vi "PTC-Restore Defaults.vi"(11 "error in (no error)":errorcluster) -> (8 "Params":T1={"Ear"=enum."Right", "Stimulus"={"Type"="", "Freq step (Hz)"=50.0, "Sampling rate (Hz)"=50000.0, "Attenuation (dB)"=20.0}, "Averages"=0, "Cal Mic Gain"=0.0, "Probe Mic Gain"=0.0, "Cal Mic Sens"=0.0, "Correction"=path ""}, 15 "error out":errorcluster)   [LabVIEW 2020]
uses:
  Typedefs/PTC-Parameters.ctl
  Common VIs/Typedefs/CAL-Stimulus.ctl
  fdd48b6a-4494-43b2-9d05-00e0dea0306e.vi
  epl-vi-lib/Utility VIs/File IO VIs/Read Write Anything/Read Anything.vi
panel:
  in  "Defaults":T1={"Ear"=enum."Right", "Stimulus"={"Type"="Chirp", "Freq step (Hz)"=50.0, "Sampling rate (Hz)"=200000.0, "Attenuation (dB)"=30.0}, "Averages"=256, "Cal Mic Gain"=40.0, "Probe Mic Gain"=40.0, "Cal Mic Sens"=-156.0, "Correction"=path ""}
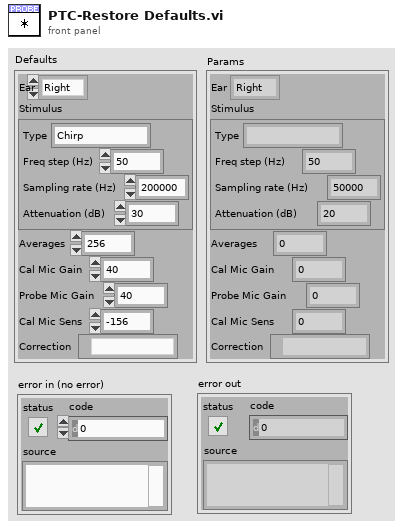
[diagram p1: front panel]
types:
  T1 = typedef "PTC-Parameters.ctl" = cluster{"Ear":enum16{"Right", "Left"}, "Stimulus":T2, "Averages":i32, "Cal Mic Gain":dbl, "Probe Mic Gain":dbl, "Cal Mic Sens":dbl, "Correction":path}
  T2 = typedef "CAL-Stimulus.ctl" = cluster{"Type":string, "Freq step (Hz)":dbl, "Sampling rate (Hz)":dbl, "Attenuation (dB)":dbl}
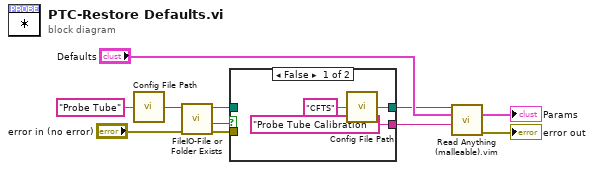
[diagram p0: block diagram]
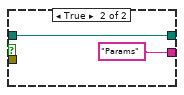
[diagram p2: hidden frame]
diagram:
  n1 = call "Config File Path.vi"("AppName"="Probe Tube") -> ("Default config file name"=w10:path)
  n2 = call "FileIO-File or Folder Exists.vi"("error in (no error)"="error in (no error)", "path"=w10) -> ("error out"=w4:errorcluster, "Exists?"=w3:bool, "dup path"=w5:path)  [unwired: 6 in, 1 out]
  n3 = case shown="False" w3 {
    tunnel: w5 -> [_ w15]
    tunnel: w4 -> [_ _]
    tunnel: ["Probe Tube Calibration" ("Section Name (Name of \"Anything\")") "Params" ("Section Name (Name of \"Anything\")")] -> w2
    tunnel: [w13 w15] -> w1
    frame False {
      n4 = call "Config File Path.vi"("AppName"="CFTS") -> ("Default config file name"=w13:path)
    }
    frame True {
    }
  }
  n5 = call "Read Anything (malleable).vim"("Config file path"=w1, "Options in"="Defaults", "Section"=w2) -> ("Options out"=→"Params":T1, "error out"=→"error out":errorcluster)  [unwired: 9 in, 2 out]
